vi "motordrivertest.vi"() -> ()   [LabVIEW 2017]
uses:
  <vilib>/Instr/_visa.llb/VISA Flush IO Buffer Mask.ctl
  <vilib>/Instr/_visa.llb/VISA Configure Serial Port (Instr).vi
panel:
  out "Motor Error Code":string
  out "error out":errorcluster
  out "Array":string[](array[string])
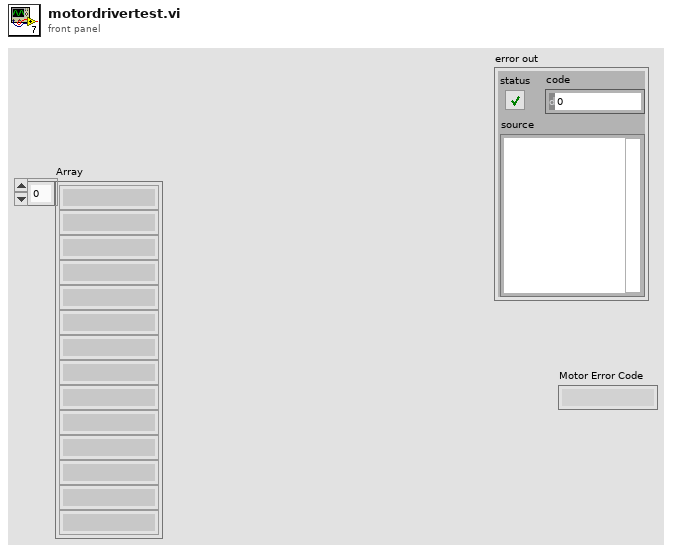
[diagram p1: front panel]
types:
  T1 = typedef "VISA Flush IO Buffer Mask.ctl" = u16
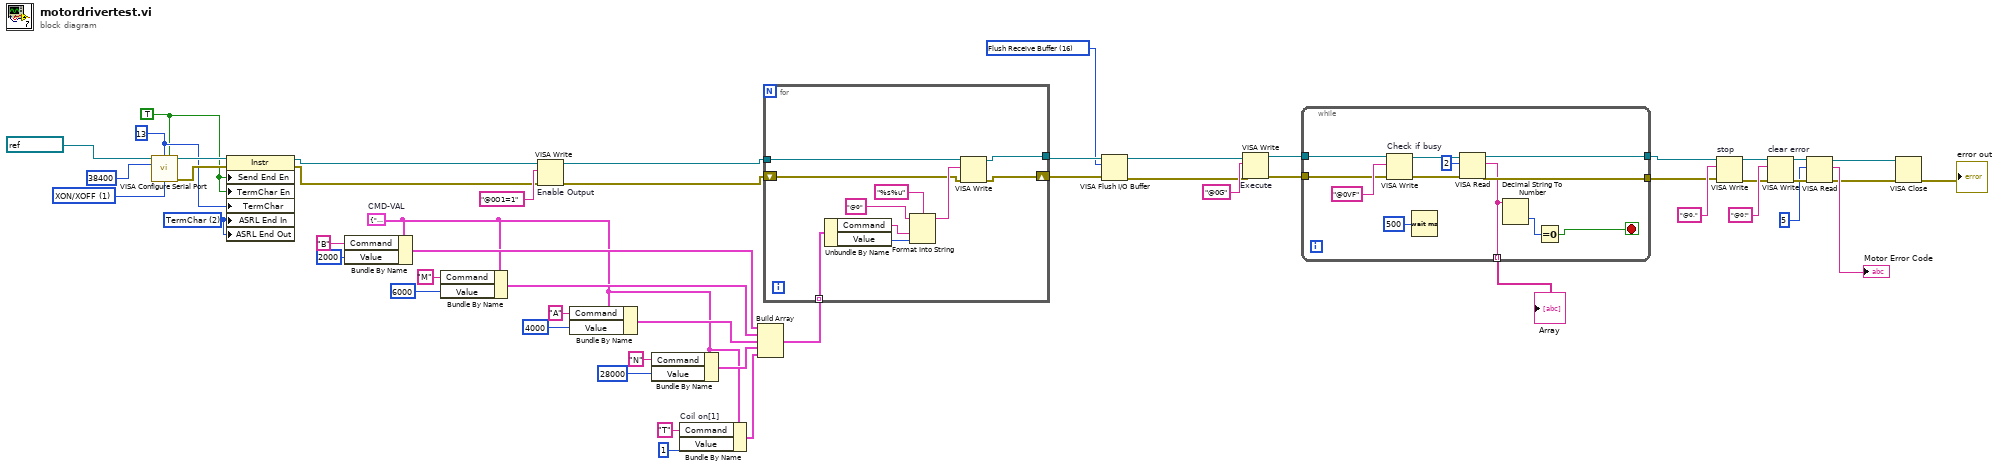
[diagram p0: block diagram]
diagram:
  w16 = u16 2 items=["None", "Last Bit", "TermChar"] ("Serial Settings:End Mode for Reads")
  w19 = T1 16 items=["Flush Receive Buffer"=16, "Write Transmit Buffer to Device"=32, "Flush Receive Buffer (No I/O)"=64, "Flush Transmit Buffer"=128] ("Mask")
  w35 = cluster{"Command":string, "Value":u32} {"Command"="A", "Value"=0}  # CMD-VAL
  w48 = u8 13 ("termination char\n(0xA = '\\n' = LF)")
  w47 = TRUE ("Enable Termination\nChar (T)")
  w50 = u16 1 items=["None", "XON/XOFF", "RTS/CTS", "XON/XOFF & RTS/CTS", "DTR/DSR", "XON/XOFF & DTR/DSR"] ("flow control (0:none)")
  n1 = call-poly "VISA Configure Serial Port"("VISA resource name"=refnum<visa-resource-name> "COM10", "termination char\n(0xA = '\\n' = LF)"=w48, "Enable Termination\nChar (T)"=w47, "baud rate (9600)"=u32 38400, "flow control (0:none)"=w50) -> ("VISA resource name out"=w51:refnum<visa-resource-name>, "error out"=w52:errorcluster)  [unwired: 9 in]
  n2 = property class="Instr"(reference=w51, error in=w52, "Send End En"=w47, "TermChar En"=w47, "TermChar"=w48, "ASRL End In"=w16, "ASRL End Out"=w16) -> (reference out=w12:refnum<visa-resource-name>, error out=w11:errorcluster)
  n3 = Bundle By Name(cluster=w35, "Command"="B", "Value"=u32 2000) -> (w39:cluster{"Command":string, "Value":u32})
  n4 = Bundle By Name(cluster=w35, "Command"="M", "Value"=u32 6000) -> (w40:cluster{"Command":string, "Value":u32})
  n5 = VISA Write "Enable Output"(VISA resource name=w12, write buffer="@0O1=1", error in (no error)=w11) -> (VISA resource name out=w14:refnum<visa-resource-name>, error out=w13:errorcluster)  [unwired: 1 out]
  n6 = Bundle By Name(cluster=w35, "Command"="A", "Value"=u32 4000) -> (w41:cluster{"Command":string, "Value":u32})
  n7 = Bundle By Name(cluster=w35, "Command"="N", "Value"=u32 28000) -> (w42:cluster{"Command":string, "Value":u32})
  n8 = Bundle By Name "Coil on[1]"(cluster=w35, "Command"="T", "Value"=u32 1) -> (w36:cluster{"Command":string, "Value":u32})
  n9 = Build Array(w39, w40, w41, w42, w36) -> (w29:cluster{"Command":string, "Value":u32}[])
  n10 = for {
    tunnel: w14 -> [w57]
    tunnel: w29 -> [w55] mode=indexing
    tunnel: [w54] -> w21
    shift-right: [w53] -> w20
    shift-left: w13 -> [w56]
    n11 = Unbundle By Name(w55) -> ("Command"=w61:string, "Value"=w62:u32)
    n12 = Format Into String(format string="%s%u", initial string="@0" ("format string"), w61, w62) -> (resulting string=w59:string)  [unwired: 1 in, 1 out]
    n13 = VISA Write(VISA resource name=w57, write buffer=w59, error in (no error)=w56) -> (VISA resource name out=w54:refnum<visa-resource-name>, error out=w53:errorcluster)  [unwired: 1 out]
  }
  n14 = VISA Flush I/O Buffer(VISA resource name=w21, mask (16)=w19, error in (no error)=w20) -> (VISA resource name out=w18:refnum<visa-resource-name>, error out=w17:errorcluster)
  n15 = VISA Write "Execute"(VISA resource name=w18, write buffer="@0G", error in (no error)=w17) -> (VISA resource name out=w27:refnum<visa-resource-name>, error out=w26:errorcluster)  [unwired: 1 out]
  n16 = while {
    tunnel: w27 -> [w72]
    tunnel: w26 -> [w73]
    tunnel: [w67] -> w24
    tunnel: [w66] -> w23
    tunnel: [w64] -> w22 mode=indexing
    stop <- w63 stop-if-true
    n17 = VISA Write "Check if busy"(VISA resource name=w72, write buffer="@0VF", error in (no error)=w73) -> (VISA resource name out=w71:refnum<visa-resource-name>, error out=w70:errorcluster)  [unwired: 1 out]
    n18 = Wait (ms)(milliseconds to wait=u32 500) -> ()  [unwired: 1 out]
    n19 = VISA Read(VISA resource name=w71, byte count=u32 2, error in (no error)=w70) -> (VISA resource name out=w67:refnum<visa-resource-name>, read buffer=w64:string, error out=w66:errorcluster)  [unwired: 1 out]
    n20 = Decimal String To Number(string=w64) -> (number=w68:i32)  [unwired: 2 in, 1 out]
    n21 = Equal To 0?(x=w68) -> (x = 0?=w63:bool)
  }
  "Array" <- w22
  n22 = VISA Write "stop"(VISA resource name=w24, write buffer="@0.", error in (no error)=w23) -> (VISA resource name out=w4:refnum<visa-resource-name>, error out=w3:errorcluster)  [unwired: 1 out]
  n23 = VISA Write "clear error"(VISA resource name=w4, write buffer="@0!", error in (no error)=w3) -> (VISA resource name out=w7:refnum<visa-resource-name>, error out=w8:errorcluster)  [unwired: 1 out]
  n24 = VISA Read(VISA resource name=w7, byte count=u32 5, error in (no error)=w8) -> (VISA resource name out=w1:refnum<visa-resource-name>, read buffer=→"Motor Error Code":string, error out=w2:errorcluster)  [unwired: 1 out]
  n25 = VISA Close(VISA resource name=w1, error in (no error)=w2) -> (error out=→"error out":errorcluster)
